vi "Initialize.vi"(8 "error in (no error)":errorcluster, 9 "Reset (Enable)":bool=TRUE, 10 "ID Query (Enable)":bool=TRUE, 11 "VISA resource name":refnum<visa-resource-name>) -> (0 "error out":errorcluster, 2 "idn string":string, 3 "VISA resource name out":refnum<visa-resource-name>)   [LabVIEW 2018, in "AWG.lvlib" / "Agilent 3352X Series.lvlib"]
doc: "Establishes communication with the instrument and optionally performs an instrument identification query and/or an instrument reset. It also places the instrument in a default state needed for other instrument driver operations. Therefore, call this VI before calling other instrument driver VIs for this instrument. Generally, you need to call the Initialize VI only once at the beginning of an application."
uses:
  Agilent 3352X Series.lvlib
  <vilib>/regexp/Match Regular Expression.xnode
panel:
  # "(c) 2011 - 2015 National Instruments.  ALL RIGHTS RESERVED."
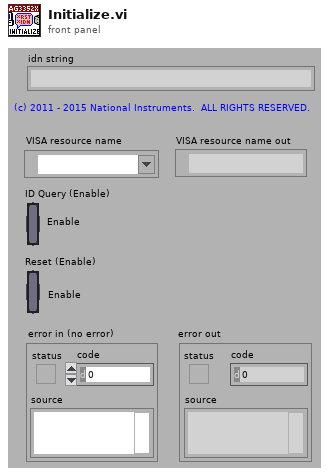
[diagram p1: front panel]
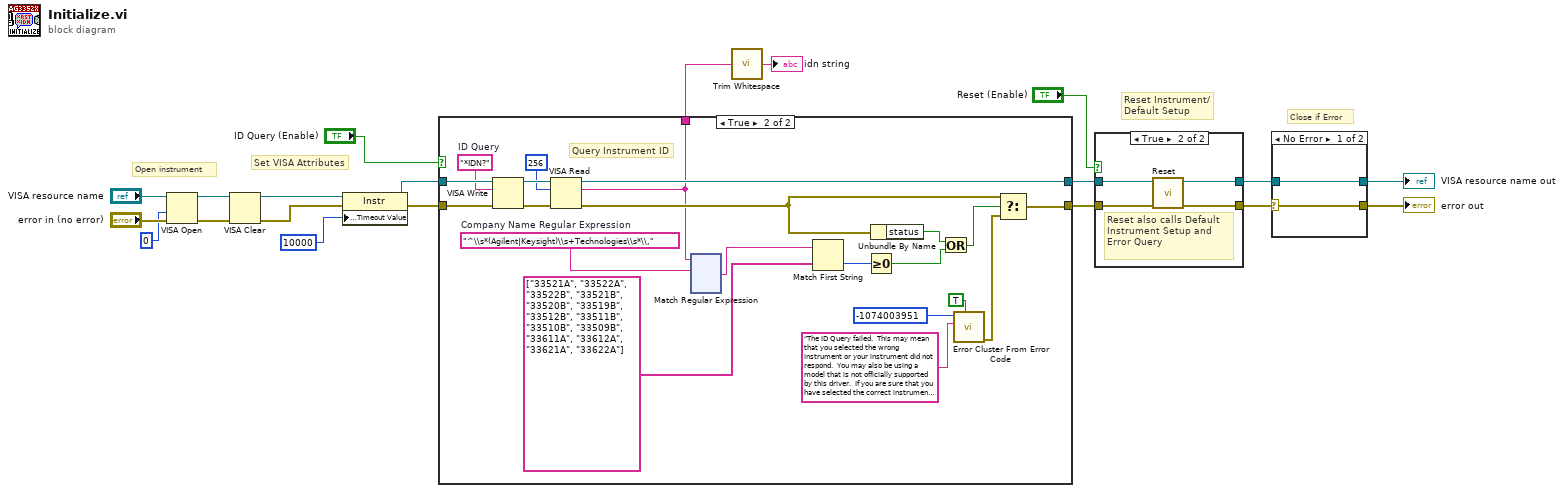
[diagram p0: block diagram]
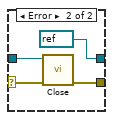
[diagram p2: hidden frame]
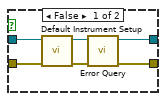
[diagram p3: hidden frame]
diagram:
  # "Set VISA Attributes"
  # "Close if Error"
  # "Reset Instrument/\nDefault Setup"
  # "Open instrument"
  n1 = VISA Open(access mode=u32 0, error in (no error)="error in (no error)", VISA resource name="VISA resource name") -> (VISA resource name=w12:refnum<visa-resource-name>, error out=w5:errorcluster)  [unwired: 2 out]
  n2 = VISA Clear(VISA resource name=w12, error in (no error)=w5) -> (VISA resource name out=w3:refnum<visa-resource-name>, error out=w4:errorcluster)
  n3 = property class="Instr"(reference=w3, error in=w4, "General Settings:Timeout Value"=u32 10000) -> (reference out=w7:refnum<visa-resource-name>, error out=w6:errorcluster)
  n4 = case shown="True" "ID Query (Enable)" {
    tunnel: [w21 w43] -> w19
    tunnel: [w22 w40] -> w20
    tunnel: w7 -> [w22 w41]
    tunnel: w6 -> [w21 w42]
    tunnel: [_ w23] -> w2
    frame False {
    }
    frame True {
      w25 = "^\\s*(Agilent|Keysight)\\s+Technologies\\s*\\,"  # Company Name Regular Expression
      w36 = "*IDN?"  # ID Query
      # "Query Instrument ID"
      n5 = VISA Write(VISA resource name=w41, write buffer=w36, error in (no error)=w42) -> (VISA resource name out=w39:refnum<visa-resource-name>, error out=w38:errorcluster)  [unwired: 1 out]
      n6 = VISA Read(VISA resource name=w39, byte count=u32 256, error in (no error)=w38) -> (VISA resource name out=w40:refnum<visa-resource-name>, read buffer=w23:string, error out=w31:errorcluster)  [unwired: 1 out]
      n7 = xnode ("Match Regular Expression")("input string"=w23, "regular expression"=w25) -> ("after match"=w24:string)  [unwired: 4 in, 4 out]
      n8 = Match First String(2:string[] ["33521A", "33522A", "33522B", "33521B", "33520B", "33519B", "33512B", "33511B", "33510B", "33509B", "33611A", "33612A", "33621A", "33622A"] ("string array"), 3:w24) -> (0:w26:i32)  [unwired: 1 out]
      n9 = Greater Or Equal To 0?(x=w26) -> (x >= 0?=w29:bool)
      n10 = Unbundle By Name(w31) -> ("status"=w30:bool)
      n11 = Or(x=w30, y=w29) -> (x .or. y?=w28:bool)
      n12 = call <vilib>:"Error Cluster From Error Code.vi"("show call chain? (False)"=TRUE, "error message (\"\")"="The ID Query failed.  This may mean that you selected the wrong instrument or your instrument did not respond.  You may also be using a model that is not officially supported by this driver.  If you are sure that you have selected the correct instrument and it is responding, try disabling the ID Query." ("Source (VI Name)"), "error code (0)"=-1074003951 ("Code")) -> ("error out"=w35:errorcluster)  [unwired: 1 in, 5 out]
      n13 = Select(t=w31, s=w28, f=w35) -> (s? t:f=w43:errorcluster)
    }
  }
  n14 = call <vilib>:"Trim Whitespace.vi"("string"=w2) -> ("trimmed string"=→"idn string":string)  [unwired: 1 in]
  n15 = case shown="True" "Reset (Enable)" {
    tunnel: w19 -> [w159 w161]
    tunnel: [w156 w164] -> w8
    tunnel: w20 -> [w160 w162]
    tunnel: [w157 w163] -> w9
    frame False {
      n16 = call "Default Instrument Setup.vi"("error in (no error)"=w159, "VISA resource name"=w160) -> ("error out"=w155:errorcluster, "VISA resource name out"=w158:refnum<visa-resource-name>)  [unwired: 8 out]
      n17 = call "Error Query.vi"("error in (no error)"=w155, "VISA resource name"=w158) -> ("error out"=w156:errorcluster, "VISA resource name out"=w157:refnum<visa-resource-name>)  [unwired: 8 out]
    }
    frame True {
      # "Reset also calls Default Instrument Setup and Error Query"
      n18 = call "Reset.vi"("error in (no error)"=w161, "VISA resource name"=w162) -> ("error out"=w164:errorcluster, "VISA resource name out"=w163:refnum<visa-resource-name>)  [unwired: 8 out]
    }
  }
  n19 = case shown="No Error" w8 {
    selector: w8 -> [w165 w168]
    tunnel: w9 -> [w166 w169]
    tunnel: [w166 refnum<visa-resource-name> refnum ("VISA resource name out")] -> w11
    tunnel: [w165 w170] -> w10
    frame No Error {
    }
    frame Error {
      n20 = call "Close.vi"("error in (no error)"=w168, "VISA resource name"=w169) -> ("error out"=w170:errorcluster)  [unwired: 9 out]
    }
  }
  "VISA resource name out" <- w11
  "error out" <- w10
